vi "unpair modules.vi"(8 "error in":errorcluster, 10 "module to pair with":refnum<class "TEC editor node.lvclass">, 11 "UDP Broadcast Editor Node in":refnum<class "TEC editor node.lvclass">) -> (0 "error out":errorcluster, 3 "UDP Broadcast Editor Node out":refnum<class "TEC editor node.lvclass">)   [LabVIEW 2013, in "TEC editor node.lvclass"]
uses:
  TEC editor node.lvclass
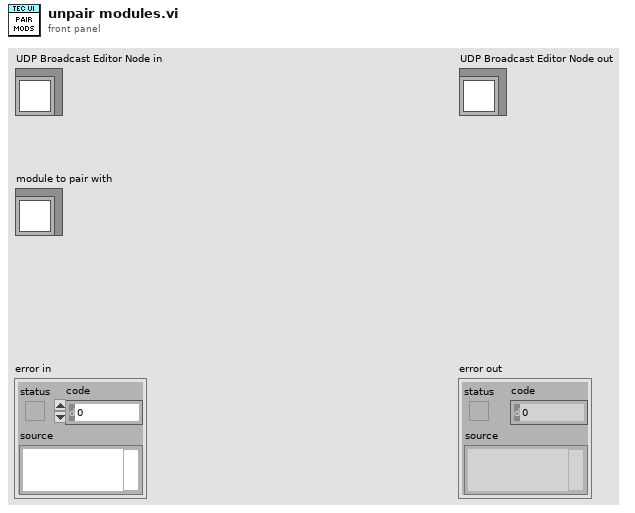
[diagram p1: front panel]
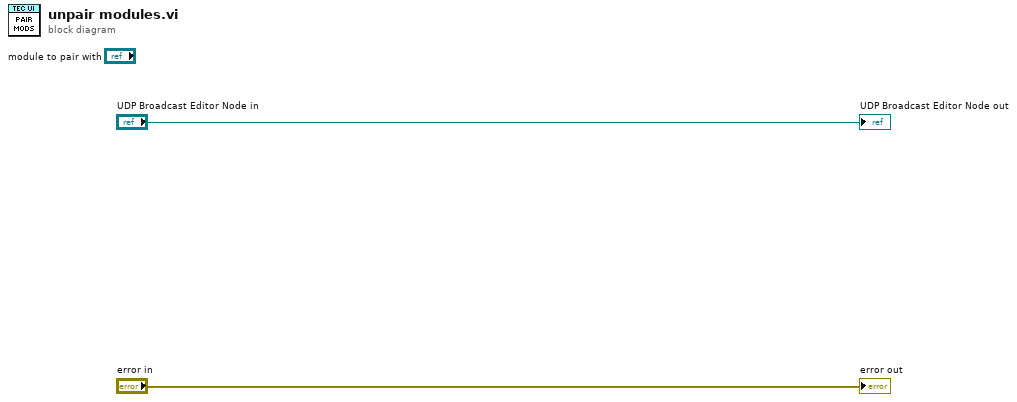
[diagram p0: block diagram]
diagram:
  "error out" <- "error in"
  "UDP Broadcast Editor Node out" <- "UDP Broadcast Editor Node in"
